vi "read_textfileByLine.vi"(11 "Byte Stream File in":refnum<file>) -> (2 "Array":dbl[](array[numeric]), 3 "Byte Stream File out":refnum<file>)   [LabVIEW 2017]
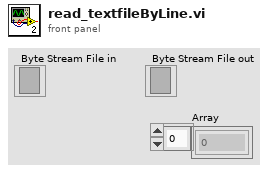
[diagram p1: front panel]
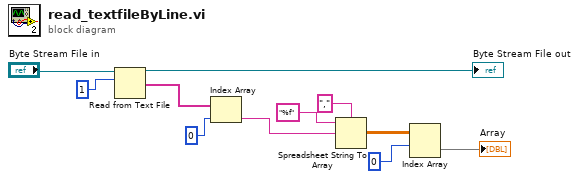
[diagram p0: block diagram]
diagram:
  n1 = Read from Text File(file (use dialog)="Byte Stream File in", count=1) -> (refnum out=→"Byte Stream File out":refnum<file>, text=w4:string[])  [unwired: 2 in, 2 out]
  n2 = Index Array(array=w4, index=0) -> (element=w11:string)
  n3 = Spreadsheet String To Array(delimiter (Tab)=",", format string="%f", spreadsheet string=w11) -> (array=w10:dbl[][])  [unwired: 1 in]
  n4 = Index Array(array=w10, index (row)=0) -> (element=→"Array":dbl[])  [unwired: 1 in]
